vi "Time_stamp.vi"() -> (0 "date/time string":string, 1 "date string":string)   [LabVIEW 2017]
panel:
  out "Error Out":errorcluster
  in  "Error In":errorcluster
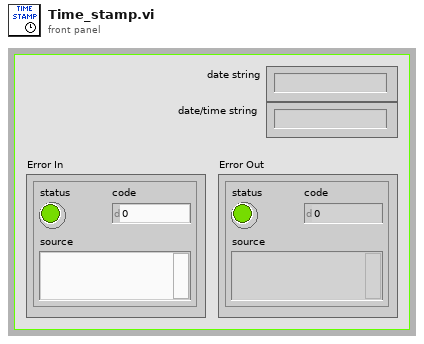
[diagram p1: front panel]
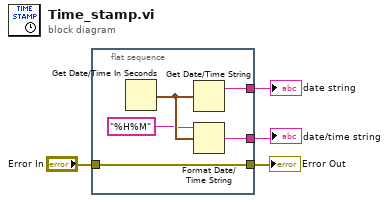
[diagram p0: block diagram]
diagram:
  n1 = flat-sequence {
    tunnel: [w9] -> w4
    tunnel: [w6] -> w3
    tunnel: "Error In" -> [w5]
    tunnel: [w5] -> w1
    frame #0 {
      n2 = Get Date/Time In Seconds() -> (seconds since 1Jan1904=w8:timestamp)
      n3 = Get Date/Time String(seconds (now)=w8) -> (date string=w9:string)  [unwired: 3 out]
      n4 = Format Date/Time String(time format string (%c)="%H%M", seconds (now)=w8) -> (date/time string=w6:string)  [unwired: 1 out]
    }
  }
  "date string" <- w4
  "date/time string" <- w3
  "Error Out" <- w1
